vi "CmdLoop.vi"(1 "ListRef":refnum<queue>) -> (0 "error out":errorcluster caption="错误输出")   [LabVIEW 2012]
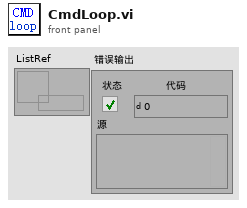
[diagram p1: front panel]
types:
  T1 = cluster{"Cmd":string, "VIref":refnum<vi>, "ListRef":refnum<queue>}
  T2 = cluster{"DeviceID":string, "Channel":string, "param1":dbl, "Operation":string}
  T3 = cluster{"ref_out":cluster{bool, "Conn. Axes out":string[]}, "ref_out":cluster{"ref_type":cluster{"MG17Motor":refnum<k7>, "MG17Motor 2":refnum<k7>, "MG17Motor 3":refnum<k7>, "MG17Motor 4":refnum<k7>, "MG17Motor 5":refnum<k7>, "MG17Motor 6":refnum<k7>}, bool[]}, "ref_out":cluster{"AG-UC2-UC8 Reference":refnum<k24>, "Instrument Key OUT":string, "Error":i32, "REDY":bool}, "ref_out":cluster{"CmdLib Out":refnum<k24>, "DeviceKey Out":string, "Device Address":i32, "REDY":bool}}
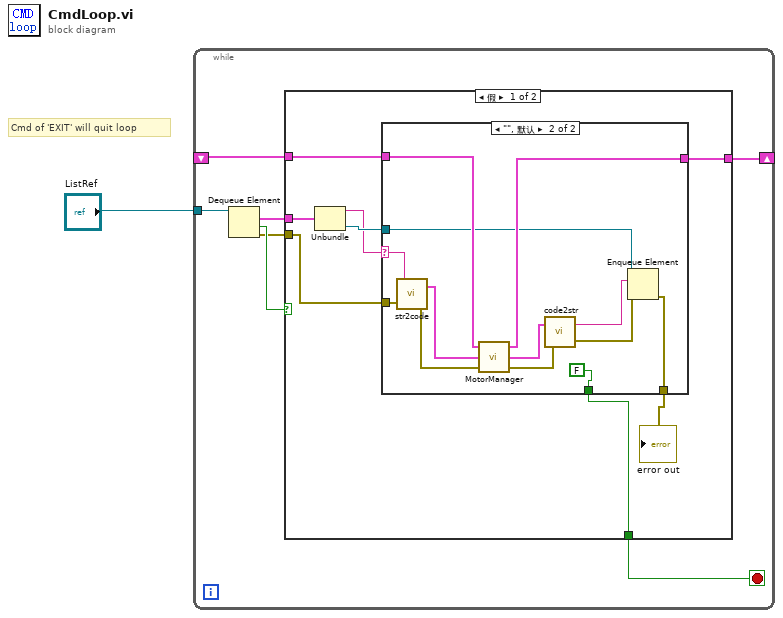
[diagram p0: block diagram]
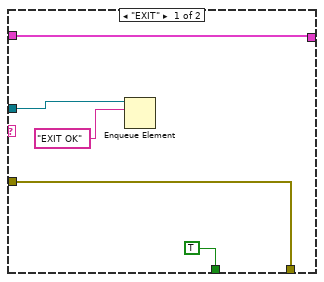
[diagram p2: hidden frame]
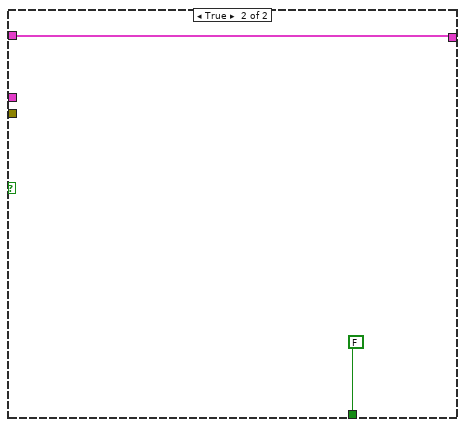
[diagram p3: hidden frame]
diagram:
  # "Cmd of 'EXIT' will quit loop"
  n1 = while {
    tunnel: "ListRef" -> [w8]
    shift-right: [w5] -> _
    shift-left: _ -> [w4]
    stop <- w2 stop-if-true
    n2 = Dequeue Element(queue=w8) -> (element=w3:T1, timed out?=w7:bool, error out=w6:errorcluster)  [unwired: 2 in, 1 out]
    n3 = case shown="假" w7 {
      tunnel: w6 -> [w12 _]
      tunnel: w4 -> [w16 w36]
      tunnel: [w15 w36] -> w5
      tunnel: w3 -> [w14 _]
      tunnel: [w9 FALSE] -> w2
      frame False {
        n4 = Unbundle(w14) -> ("Cmd"=w10:string, "ListRef"=w13:refnum<queue>)  [unwired: 1 out]
        n5 = case shown="\"\", 默认" w10 {
          selector: w10 -> [_ w23]
          tunnel: w16 -> [w21 w34]
          tunnel: [w21 w33] -> w15
          tunnel: w13 -> [w17 w29]
          tunnel: w12 -> [w20 w28]
          tunnel: [w20 w24] -> w11
          tunnel: [TRUE FALSE] -> w9
          frame "EXIT" {
            n6 = Enqueue Element(queue=w17, element="EXIT OK" ("元素")) -> ()  [unwired: 2 in, 3 out]
          }
          frame "", Default {
            n7 = call "str2code.vi"("错误输入"=w28, "input"=w23) -> ("error out"=w27:errorcluster, "Output"=w32:T2)
            n8 = call "MotorManager.vi"("error in (no error)"=w27, "Input"=w32, "ref_in"=w34) -> ("error out"=w26:errorcluster, "Output"=w31:T2, "ref_out"=w33:T3)
            n9 = call "code2str.vi"("错误输入"=w26, "input"=w31) -> ("error out"=w25:errorcluster, "output"=w30:string)
            n10 = Enqueue Element(queue=w29, element=w30, error in (no error)=w25) -> (error out=w24:errorcluster)  [unwired: 1 in, 2 out]
          }
        }
        "error out" <- w11
      }
      frame True {
      }
    }
  }
